vi "Panel-OIM-ShutterMagliteCornerCube.vi"(0 "error in":errorcluster caption="entrée d'erreur") -> (3 "error out":errorcluster caption="sortie d'erreur")   [LabVIEW 2009]
panel:
  in  "PI2 Cube":bool
  in  "PI1 Cube":bool
  in  "Stop":bool
  in  "PI2 INIT":bool
  in  "PI1 INIT":bool
  in  "PI2 Maglite":i32(knob) min=0 max=90 step=1 scale=0.0..83.0
  in  "PI1 Maglite":i32(knob) min=0 max=90 step=1 scale=0.0..83.0
  in  "PI2 Shutter":bool
  in  "PI1 Shutter":bool
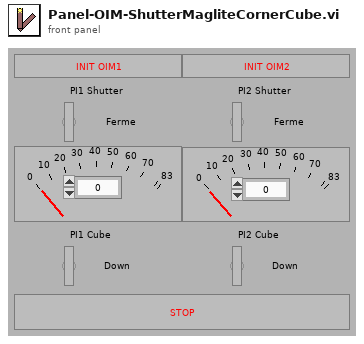
[diagram p1: front panel]
types:
  T1 = typedef "SourceStatus.ctl" = cluster{"Managed?":bool, "Intensity":i32}
  T2 = typedef "MotorStatus.ctl" = cluster{"Managed?":bool, "Position":i32, "Name":string, "Status":enum16{"OFF", "IDLE", "MOVING", "HOMING"}}
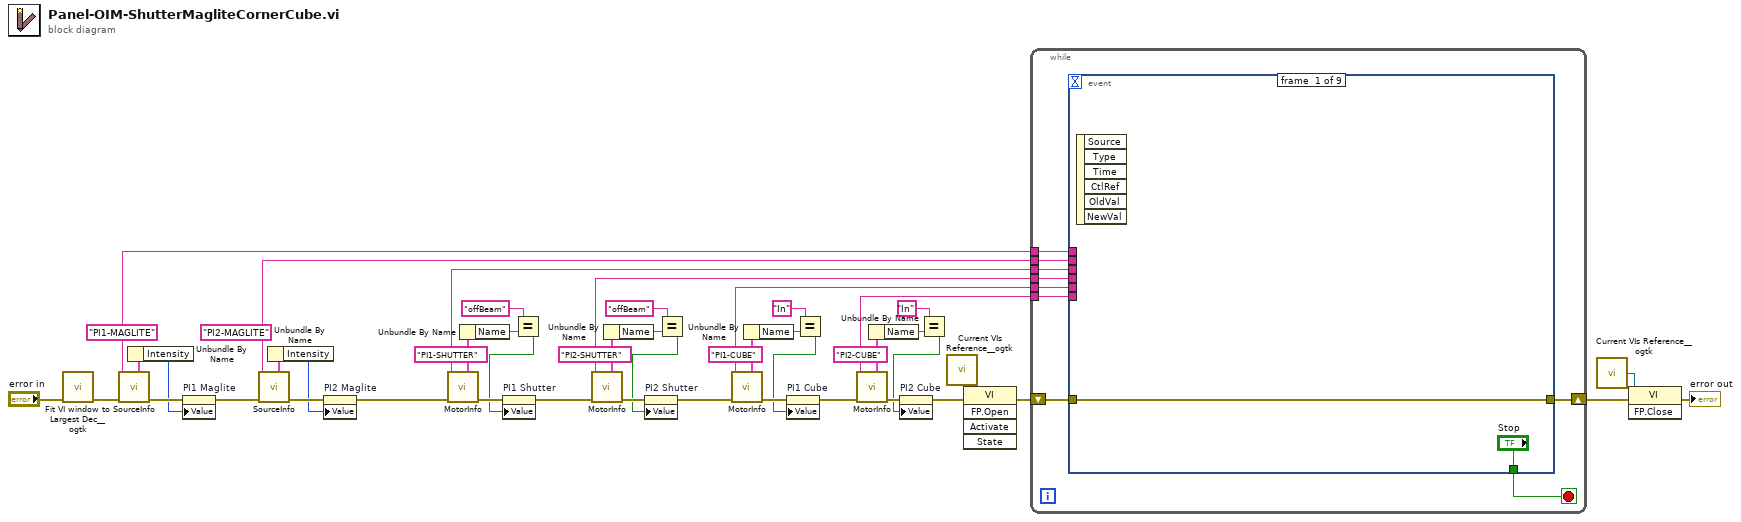
[diagram p0: block diagram]
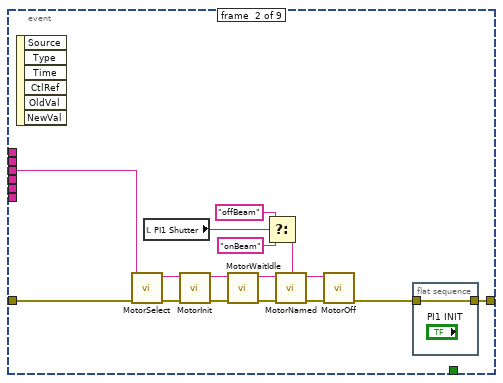
[diagram p2: hidden frame]
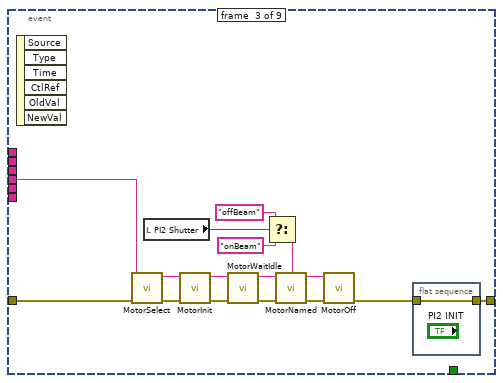
[diagram p3: hidden frame]
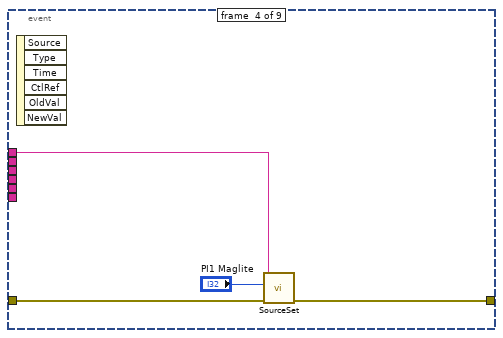
[diagram p4: hidden frame]
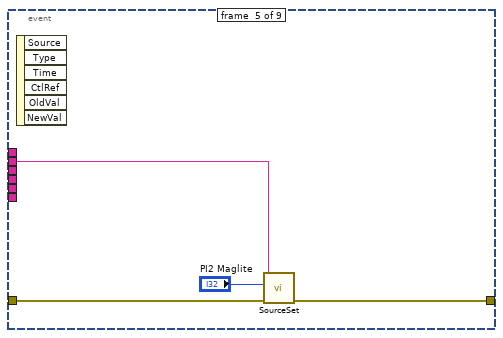
[diagram p5: hidden frame]
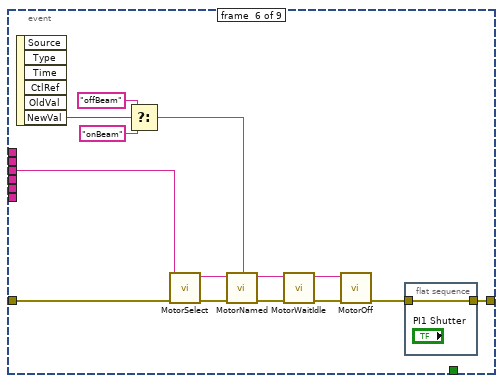
[diagram p6: hidden frame]
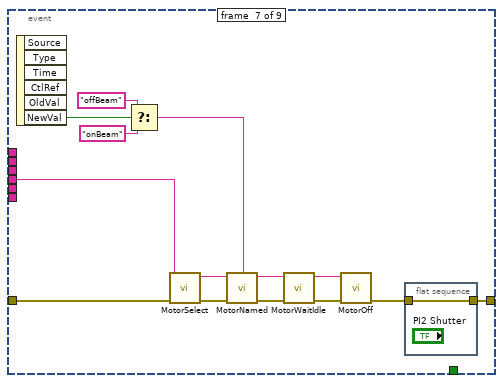
[diagram p7: hidden frame]
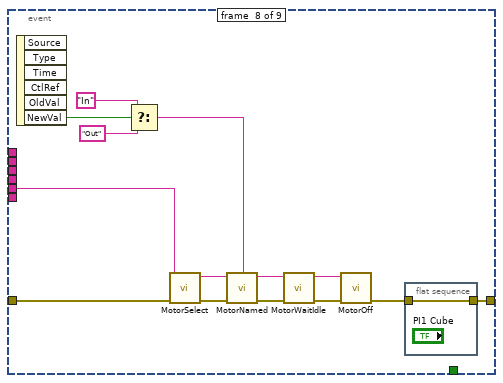
[diagram p8: hidden frame]
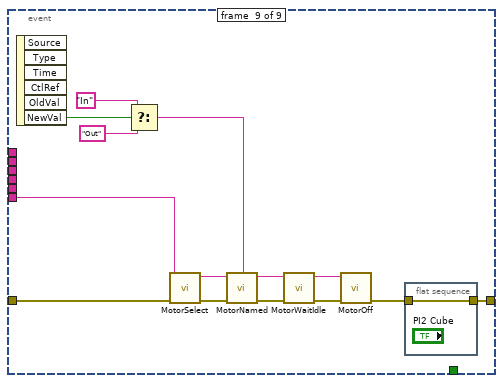
[diagram p9: hidden frame]
diagram:
  w12 = "PI2-CUBE" ("Motor in")
  w17 = "PI1-CUBE" ("Motor in")
  w24 = "PI2-MAGLITE"
  w25 = "PI1-MAGLITE"
  w4 = "PI2-SHUTTER"
  w5 = "PI1-SHUTTER"
  n1 = call <userlib>:"Fit VI window to Largest Dec__ogtk.vi"("error in (no error)"="error in") -> ("error out"=w41:errorcluster)  [unwired: 2 in, 4 out]
  n2 = call "SourceInfo.vi"("error in (no error)"=w41, "Source"=w25) -> ("error out"=w39:errorcluster, "SourceStatus"=w40:T1)  [unwired: 6 out]
  n3 = Unbundle By Name(w40) -> ("Intensity"=w38:i32)
  n4 = property on="PI1 Maglite" class="Bouton rotatif (strict)"(error in=w39, "Value"=w38) -> (error out=w36:errorcluster)  [unwired: 1 in, 1 out]
  n5 = call "SourceInfo.vi"("error in (no error)"=w36, "Source"=w24) -> ("error out"=w35:errorcluster, "SourceStatus"=w37:T1)  [unwired: 6 out]
  n6 = Unbundle By Name(w37) -> ("Intensity"=w34:i32)
  n7 = property on="PI2 Maglite" class="Bouton rotatif (strict)"(error in=w35, "Value"=w34) -> (error out=w2:errorcluster)  [unwired: 1 in, 1 out]
  n8 = call "MotorInfo.vi"("error in (no error)"=w2, "Motor"=w5) -> ("error out"=w33:errorcluster, "Axis status"=w45:T2)  [unwired: 6 out]
  n9 = Unbundle By Name(w45) -> ("Name"=w32:string)
  n10 = Equal?(x="offBeam", y=w32) -> (x = y?=w31:bool)
  n11 = property on="PI1 Shutter" class="Bool (strict)"(error in=w33, "Value"=w31) -> (error out=w3:errorcluster)  [unwired: 1 in, 1 out]
  n12 = call "MotorInfo.vi"("error in (no error)"=w3, "Motor"=w4) -> ("error out"=w27:errorcluster, "Axis status"=w44:T2)  [unwired: 6 out]
  n13 = Unbundle By Name(w44) -> ("Name"=w28:string)
  n14 = Equal?(x="offBeam", y=w28) -> (x = y?=w26:bool)
  n15 = property on="PI2 Shutter" class="Bool (strict)"(error in=w27, "Value"=w26) -> (error out=w23:errorcluster)  [unwired: 1 in, 1 out]
  n16 = call "MotorInfo.vi"("error in (no error)"=w23, "Motor"=w17) -> ("error out"=w19:errorcluster, "Axis status"=w22:T2)  [unwired: 6 out]
  n17 = Unbundle By Name(w22) -> ("Name"=w20:string)
  n18 = Equal?(x="In", y=w20) -> (x = y?=w18:bool)
  n19 = property on="PI1 Cube" class="Bool (strict)"(error in=w19, "Value"=w18) -> (error out=w13:errorcluster)  [unwired: 1 in, 1 out]
  n20 = call "MotorInfo.vi"("error in (no error)"=w13, "Motor"=w12) -> ("error out"=w11:errorcluster, "Axis status"=w14:T2)  [unwired: 6 out]
  n21 = Unbundle By Name(w14) -> ("Name"=w16:string)
  n22 = Equal?(x="In", y=w16) -> (x = y?=w10:bool)
  n23 = property on="PI2 Cube" class="Bool (strict)"(error in=w11, "Value"=w10) -> (error out=w7:errorcluster)  [unwired: 1 in, 1 out]
  n24 = call <userlib>:"Current VIs Reference__ogtk.vi"() -> ("Current VI's reference"=w9:refnum<vi>)  [unwired: 5 out]
  n25 = invoke class="VI" method="FP.Open"(reference=w9, error in=w7) -> (error out=w6:errorcluster)  [unwired: 3 in, 4 out]
  n26 = while {
    tunnel: w25 -> [w52]
    tunnel: w24 -> [w51]
    tunnel: w5 -> [w50]
    tunnel: w4 -> [w49]
    tunnel: w17 -> [w48]
    tunnel: w12 -> [w47]
    shift-right: [w54] -> w1
    shift-left: w6 -> [w46]
    stop <- w53 stop-if-true
    n27 = event shown="[2] \"PI2 INIT\": Value Change" {
      selector: _ -> [_ _ _ _ _ _ _ _ _]
      dyn-events: _ -> [_ _ _ _ _ _ _ _ _]
      timeout: _ -> [_ _ _ _ _ _ _ _ _]
      tunnel: [w55 w70 w89 w94 w98 w112 w127 w142 w157] -> w54
      tunnel: ["Stop" _ _ _ _ _ _ _ _] -> w53
      tunnel: w52 -> [_ _ _ w93 _ _ _ _ _]
      tunnel: w51 -> [_ _ _ _ w96 _ _ _ _]
      tunnel: w50 -> [_ w65 _ _ _ w100 _ _ _]
      tunnel: w49 -> [_ _ w79 _ _ _ w114 _ _]
      tunnel: w48 -> [_ _ _ _ _ _ _ w130 _]
      tunnel: w47 -> [_ _ _ _ _ _ _ _ w145]
      tunnel: w46 -> [w55 w63 w81 w91 w95 w102 w117 w129 w144]
      event #0 {
        n28 = event-data() -> ()  [unwired: 7 out]
      }
      event #1 {
        n29 = event-data() -> ()  [unwired: 7 out]
        n30 = call "MotorSelect.vi"("Motor"=w65, "error in (no error)"=w63) -> ("Motor out"=w64:string, "error out"=w62:errorcluster)  [unwired: 6 out]
        n31 = local read "PI1 Shutter"() -> (w66:bool)
        n32 = call "MotorInit.vi"("Motor"=w64, "error in (no error)"=w62) -> ("Motor out"=w71:string, "error out"=w72:errorcluster)  [unwired: 6 out]
        n33 = call "MotorWaitIdle.vi"("Motor"=w71, "error in (no error)"=w72) -> ("Motor out"=w60:string, "error out"=w61:errorcluster)  [unwired: 6 out]
        n34 = Select(t="offBeam", s=w66, f="onBeam") -> (s? t:f=w69:string)
        n35 = call "MotorNamed.vi"("Name"=w69, "Motor in"=w60, "error in (no error)"=w61) -> ("Motor out"=w57:string, "error out"=w59:errorcluster)  [unwired: 5 out]
        n36 = call "MotorOff.vi"("Motor"=w57, "error in (no error)"=w59) -> ("error out"=w58:errorcluster)  [unwired: 7 out]
        n37 = flat-sequence {
          tunnel: [w73] -> w70
          tunnel: w58 -> [w73]
          frame #0 {
          }
        }
      }
      event #2 {
        n38 = event-data() -> ()  [unwired: 7 out]
        n39 = call "MotorSelect.vi"("Motor"=w79, "error in (no error)"=w81) -> ("Motor out"=w78:string, "error out"=w84:errorcluster)  [unwired: 6 out]
        n40 = local read "PI2 Shutter"() -> (w86:bool)
        n41 = call "MotorInit.vi"("Motor"=w78, "error in (no error)"=w84) -> ("Motor out"=w77:string, "error out"=w85:errorcluster)  [unwired: 6 out]
        n42 = call "MotorWaitIdle.vi"("Motor"=w77, "error in (no error)"=w85) -> ("Motor out"=w76:string, "error out"=w83:errorcluster)  [unwired: 6 out]
        n43 = Select(t="offBeam", s=w86, f="onBeam") -> (s? t:f=w74:string)
        n44 = call "MotorNamed.vi"("Name"=w74, "Motor in"=w76, "error in (no error)"=w83) -> ("Motor out"=w75:string, "error out"=w82:errorcluster)  [unwired: 5 out]
        n45 = call "MotorOff.vi"("Motor"=w75, "error in (no error)"=w82) -> ("error out"=w80:errorcluster)  [unwired: 7 out]
        n46 = flat-sequence {
          tunnel: [w90] -> w89
          tunnel: w80 -> [w90]
          frame #0 {
          }
        }
      }
      event #3 {
        n47 = event-data() -> ()  [unwired: 7 out]
        n48 = call "SourceSet.vi"("Source"=w93, "Intensity"="PI1 Maglite", "error in (no error)"=w91) -> ("error out"=w94:errorcluster)  [unwired: 6 out]
      }
      event #4 {
        n49 = event-data() -> ()  [unwired: 7 out]
        n50 = call "SourceSet.vi"("Source"=w96, "Intensity"="PI2 Maglite", "error in (no error)"=w95) -> ("error out"=w98:errorcluster)  [unwired: 6 out]
      }
      event #5 {
        n51 = event-data() -> ("NewVal"=w111:bool)  [unwired: 6 out]
        n52 = Select(t="offBeam", s=w111, f="onBeam") -> (s? t:f=w99:string)
        n53 = call "MotorSelect.vi"("Motor"=w100, "error in (no error)"=w102) -> ("Motor out"=w107:string, "error out"=w108:errorcluster)  [unwired: 6 out]
        n54 = call "MotorNamed.vi"("Name"=w99, "Motor in"=w107, "error in (no error)"=w108) -> ("Motor out"=w104:string, "error out"=w106:errorcluster)  [unwired: 5 out]
        n55 = call "MotorWaitIdle.vi"("Motor"=w104, "error in (no error)"=w106) -> ("Motor out"=w103:string, "error out"=w105:errorcluster)  [unwired: 6 out]
        n56 = call "MotorOff.vi"("Motor"=w103, "error in (no error)"=w105) -> ("error out"=w101:errorcluster)  [unwired: 7 out]
        n57 = flat-sequence {
          tunnel: [w113] -> w112
          tunnel: w101 -> [w113]
          frame #0 {
          }
        }
      }
      event #6 {
        n58 = event-data() -> ("NewVal"=w126:bool)  [unwired: 6 out]
        n59 = Select(t="offBeam", s=w126, f="onBeam") -> (s? t:f=w115:string)
        n60 = call "MotorSelect.vi"("Motor"=w114, "error in (no error)"=w117) -> ("Motor out"=w122:string, "error out"=w123:errorcluster)  [unwired: 6 out]
        n61 = call "MotorNamed.vi"("Name"=w115, "Motor in"=w122, "error in (no error)"=w123) -> ("Motor out"=w119:string, "error out"=w121:errorcluster)  [unwired: 5 out]
        n62 = call "MotorWaitIdle.vi"("Motor"=w119, "error in (no error)"=w121) -> ("Motor out"=w118:string, "error out"=w120:errorcluster)  [unwired: 6 out]
        n63 = call "MotorOff.vi"("Motor"=w118, "error in (no error)"=w120) -> ("error out"=w116:errorcluster)  [unwired: 7 out]
        n64 = flat-sequence {
          tunnel: [w128] -> w127
          tunnel: w116 -> [w128]
          frame #0 {
          }
        }
      }
      event #7 {
        n65 = event-data() -> ("NewVal"=w141:bool)  [unwired: 6 out]
        n66 = Select(t="In", s=w141, f="Out") -> (s? t:f=w138:string)
        n67 = call "MotorSelect.vi"("Motor"=w130, "error in (no error)"=w129) -> ("Motor out"=w136:string, "error out"=w137:errorcluster)  [unwired: 6 out]
        n68 = call "MotorNamed.vi"("Name"=w138, "Motor in"=w136, "error in (no error)"=w137) -> ("Motor out"=w132:string, "error out"=w135:errorcluster)  [unwired: 5 out]
        n69 = call "MotorWaitIdle.vi"("Motor"=w132, "error in (no error)"=w135) -> ("Motor out"=w131:string, "error out"=w134:errorcluster)  [unwired: 6 out]
        n70 = call "MotorOff.vi"("Motor"=w131, "error in (no error)"=w134) -> ("error out"=w133:errorcluster)  [unwired: 7 out]
        n71 = flat-sequence {
          tunnel: [w143] -> w142
          tunnel: w133 -> [w143]
          frame #0 {
          }
        }
      }
      event #8 {
        n72 = event-data() -> ("NewVal"=w156:bool)  [unwired: 6 out]
        n73 = Select(t="In", s=w156, f="Out") -> (s? t:f=w153:string)
        n74 = call "MotorSelect.vi"("Motor"=w145, "error in (no error)"=w144) -> ("Motor out"=w151:string, "error out"=w152:errorcluster)  [unwired: 6 out]
        n75 = call "MotorNamed.vi"("Name"=w153, "Motor in"=w151, "error in (no error)"=w152) -> ("Motor out"=w147:string, "error out"=w150:errorcluster)  [unwired: 5 out]
        n76 = call "MotorWaitIdle.vi"("Motor"=w147, "error in (no error)"=w150) -> ("Motor out"=w146:string, "error out"=w149:errorcluster)  [unwired: 6 out]
        n77 = call "MotorOff.vi"("Motor"=w146, "error in (no error)"=w149) -> ("error out"=w148:errorcluster)  [unwired: 7 out]
        n78 = flat-sequence {
          tunnel: [w158] -> w157
          tunnel: w148 -> [w158]
          frame #0 {
          }
        }
      }
    }
  }
  n79 = call <userlib>:"Current VIs Reference__ogtk.vi"() -> ("Current VI's reference"=w43:refnum<vi>)  [unwired: 5 out]
  n80 = invoke class="VI" method="FP.Close"(reference=w43, error in=w1) -> (error out=→"error out":errorcluster)  [unwired: 1 in, 2 out]
